vi "user input.vi"(8 "error in":errorcluster) -> (0 "error out":errorcluster, 3 "Inputs from system":T1)   [LabVIEW 2013, in "My Awesome Control Modules runtime.lvclass"]
uses:
  My Awesome Control Modules runtime.lvclass
  input user data.ctl
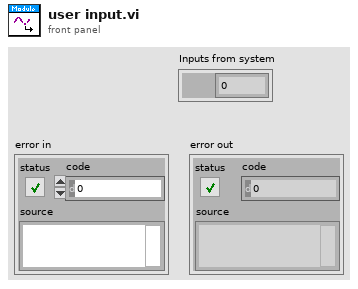
[diagram p1: front panel]
types:
  T1 = typedef "My Awesome Control Modules runtime.lvclass/input user data.ctl" = cluster{"asd":dbl}
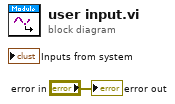
[diagram p0: block diagram]
diagram:
  "error out" <- "error in"
